vi "Read Shift Registers.vi"(8 "error in (no error)":errorcluster, 11 "Loop in":refnum<class "Loop.lvclass">) -> (0 "error out":errorcluster, 2 "Shift Registers":T1[](array[typedef]), 3 "Loop out":refnum<class "Loop.lvclass">)   [LabVIEW 2025, in "Loop.lvclass"]
uses:
  Loop.lvclass
  Controls/Shift Register.ctl
  Controls/Terminal.ctl
  Loop.lvclass/Loop.ctl
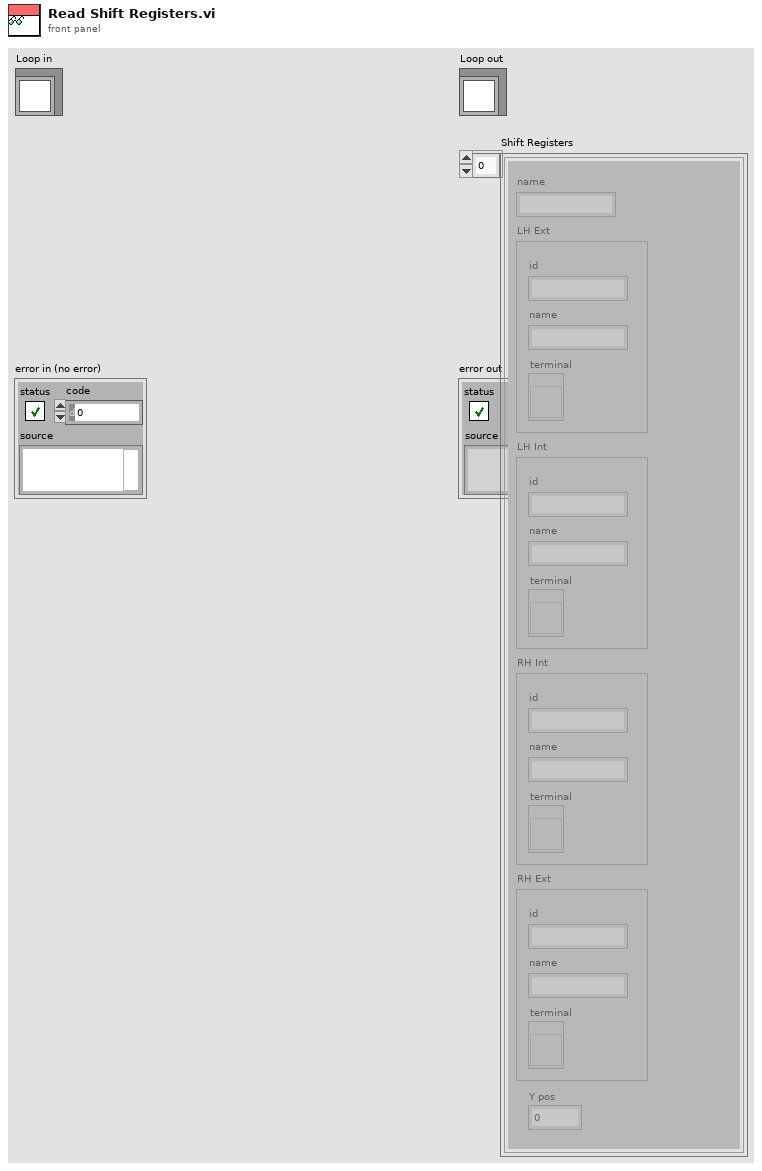
[diagram p1: front panel]
types:
  T1 = typedef "Shift Register.ctl" = cluster{"name":string, "LH Ext":T2, "LH Int":T2, "RH Int":T2, "RH Ext":T2, "Y pos":u32}
  T2 = typedef "Terminal.ctl" = cluster{"id":string, "name":string, "terminal":refnum<vi>}
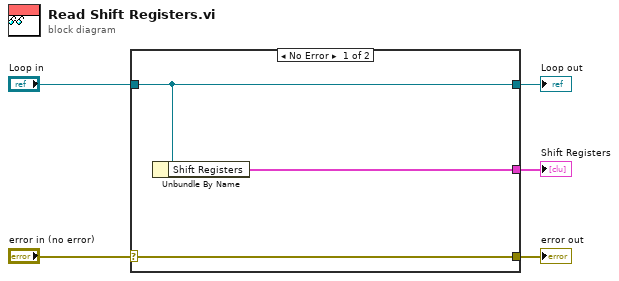
[diagram p0: block diagram]
diagram:
  n1 = case shown="No Error" "error in (no error)" {
    selector: "error in (no error)" -> [w8 w9]
    tunnel: [w8 w9] -> w4
    tunnel: [w7 w10] -> w2
    tunnel: "Loop in" -> [w7 w10]
    tunnel: [w6 _] -> w1
    frame No Error {
      n2 = Unbundle By Name(w7) -> ("Shift Registers"=w6:T1[])
    }
    frame Error {
    }
  }
  "error out" <- w4
  "Loop out" <- w2
  "Shift Registers" <- w1
